vi "Stop Core.vi"(10 "final error code":i32, 11 "[V] Main UI in":refnum<class "[V] Main UI.lvclass">) -> (3 "[V] Main UI out":refnum<class "[V] Main UI.lvclass">)   [LabVIEW 2020, in "[V] Main UI.lvlib" / "[V] Main UI.lvclass"]
doc: "(<B>Filename</B>: Actor Framework.lvlib:Actor.lvclass:Stop Core.vi)\n\nDefines what the actor does before it stops. Use the <B>final error code</B> input to determine whether the actor shut down in response to an error.\n\nBy default, this method passes the Stop message along to all auto-stop nested actors. A descendant class may override this method to define additional behavior, such as shutting down any processes the actor initiated in its override of the Actor Core method."
uses:
  [V] Main UI.lvclass
  MVVM Framework/MVVM Abstruct View/MVVM Abstruct View/MVVM Abstruct View.lvclass
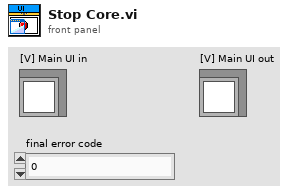
[diagram p1: front panel]
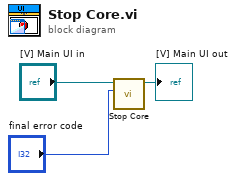
[diagram p0: block diagram]
diagram:
  n1 = call-parent "Stop Core.vi"("final error code"="final error code", "Abstruct View in"="[V] Main UI in") -> ("Abstruct View out"=→"[V] Main UI out":refnum<class "[V] Main UI.lvclass">)  [unwired: 9 in]
